vi "Data Sent.vi"(5 "Component ID":u8, 7 "FPGA Interface":refnum<class "FPGA Interface.lvclass">, 8 "error in (no error)":errorcluster, 10 "Tx SubAddress (1-30)":u16, 11 "Remote Terminal in":refnum<class "Remote Terminal.lvclass">) -> (0 "error out":errorcluster, 2 "Data Transmitted?":bool)   [LabVIEW 2020, in "BCI-1553 API.lvlib" / "Remote Terminal.lvclass"]
doc: "Checks IC memory to determine if a transmit subaddress has sent any data. This flag will latch high after the first time the subaddress transmits data. Call the 'Clear Data Sent Flag' method to reset the flag."
uses:
  Remote Terminal.lvclass
  Dependencies/FPGA Interface/FPGA Interface.lvclass
  Remote Terminal.lvclass/Remote Terminal.ctl
panel:
  out "debug":u16 format="%04x"
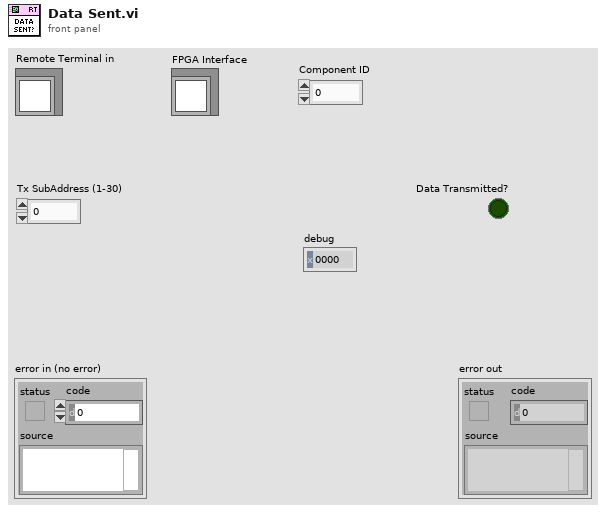
[diagram p1: front panel]
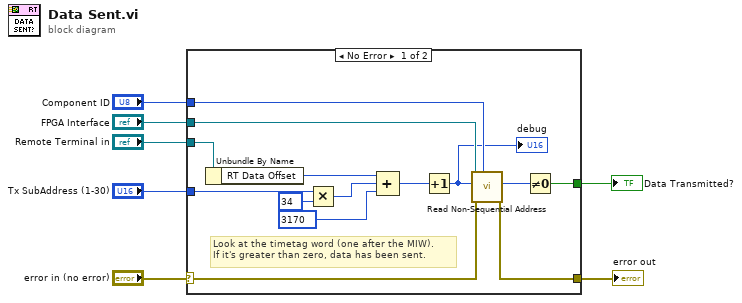
[diagram p0: block diagram]
diagram:
  n1 = case shown="No Error" "error in (no error)" {
    selector: "error in (no error)" -> [w9 w22]
    tunnel: [w10 w22] -> w6
    tunnel: "Remote Terminal in" -> [w19 _]
    tunnel: "FPGA Interface" -> [w21 _]
    tunnel: "Component ID" -> [w20 _]
    tunnel: "Tx SubAddress (1-30)" -> [w16 _]
    tunnel: [w11 _] -> w1
    frame No Error {
      # "Look at the timetag word (one after the MIW).\nIf it's greater than zero, data has been sent."
      n2 = Unbundle By Name(w19) -> ("RT Data Offset"=w14:u16)
      n3 = Multiply(x=w16, y=u16 34 ("Address")) -> (x*y=w15:u16)
      n4 = Compound Arithmetic op=ADD(w14, w15, u16 3170 ("Address")) -> (w13:u16)
      n5 = Increment(x=w13) -> (x+1=w8:u16)
      "debug" <- w8
      n6 = call-dynamic "Read Non-Sequential Address.vi"("Target IC (1-8)"=w20, "error in (no error)"=w9, "Address"=w8, "FPGA Interface in"=w21) -> ("error out"=w10:errorcluster, "Data"=w12:u16)  [unwired: 6 in]
      n7 = Not Equal To 0?(x=w12) -> (x != 0?=w11:bool)
    }
    frame Error {
    }
  }
  "error out" <- w6
  "Data Transmitted?" <- w1
